vi "Run.vi"(8 "error in (no error)":errorcluster, 11 "LUnit Test Case V2 in":refnum<class "LUnit Test Case V2.lvclass">) -> (0 "error out":errorcluster, 2 "Results":T1[](array[typedef]))   [LabVIEW 2020, in "LUnit Test Case V2.lvclass"]
uses:
  LUnit Test Case V2.lvclass
  Result/Result.ctl
  Result/Status.ctl
  Result/Type.ctl
  LUnit Test Case V2.lvclass/LUnit Test Case V2.ctl
  Result/Result.lvlib
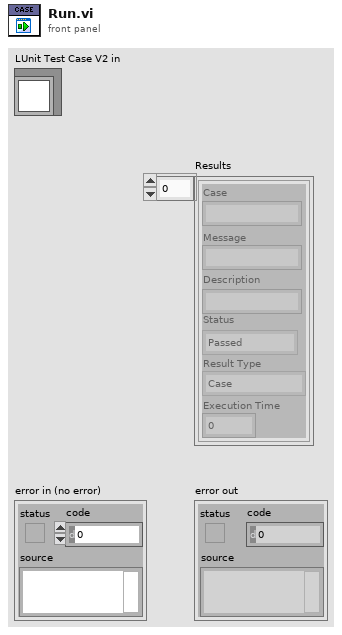
[diagram p1: front panel]
types:
  T1 = typedef "Result.lvlib/Result.ctl" = cluster{"Case":string, "Message":string, "Description":string, "Status":T2, "Result Type":T3, "Execution Time":dbl}
  T2 = typedef "Result.lvlib/Status.ctl" = enum16{"Passed", "Failed", "Error", "Skipped", "Setup Error", "Broken", "Teardown Error"}
  T3 = typedef "Result.lvlib/Type.ctl" = enum16{"Method", "Case", "Suite", "Pass", "Fail", "Skip", "Pass if", "Fail if", "Pass if Error", "Fail if Error", "Pass if Equal", "Fail if Equal"}
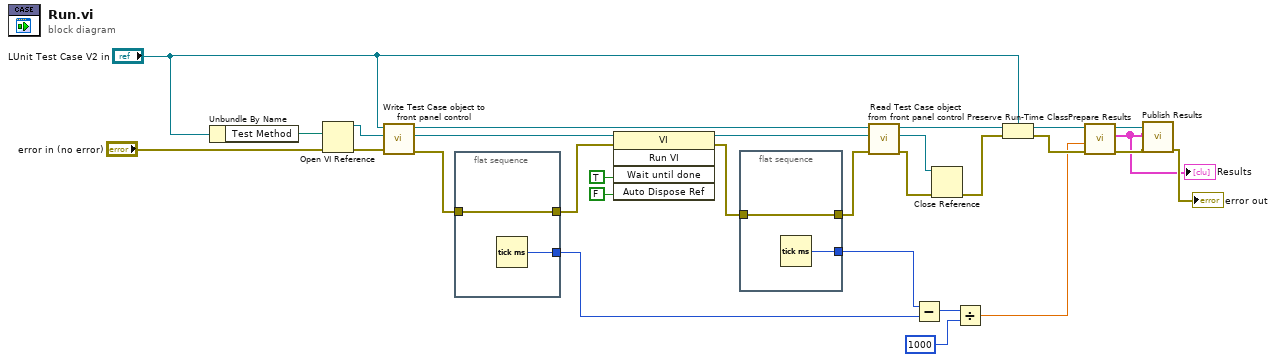
[diagram p0: block diagram]
diagram:
  n1 = Unbundle By Name("LUnit Test Case V2 in") -> ("Test Method"=w20:path)
  n2 = Open VI Reference(vi path=w20, error in (no error)="error in (no error)") -> (vi reference=w22:refnum<vi>, error out=w21:errorcluster)  [unwired: 4 in]
  n3 = call "Write Test Case object to front panel control.vi"("error in (no error)"=w21, "VI Refnum"=w22, "Test Case in"="LUnit Test Case V2 in") -> ("error out"=w13:errorcluster, "VI Refnum out"=w18:refnum<vi>, "Test Case out"=w15:refnum<class "LUnit Test Case V2.lvclass">)  [unwired: 6 in]
  n4 = flat-sequence {
    tunnel: w13 -> [w31]
    tunnel: [w31] -> w12
    tunnel: [w30] -> w8
    frame #0 {
      n5 = Tick Count (ms)() -> (millisecond timer value=w30:u32)
    }
  }
  n6 = invoke class="VI" method="Run VI"(reference=w18, error in=w12, "Wait until done"=TRUE ("Wait Until Done"), "Auto Dispose Ref"=FALSE ("Auto Dispose Reference")) -> (reference out=w19:refnum<vi>, error out=w11:errorcluster)  [unwired: 1 in, 3 out]
  n7 = flat-sequence {
    tunnel: w11 -> [w33]
    tunnel: [w33] -> w10
    tunnel: [w32] -> w9
    frame #0 {
      n8 = Tick Count (ms)() -> (millisecond timer value=w32:u32)
    }
  }
  n9 = call "Read Test Case object from front panel control.vi"("error in (no error)"=w10, "VI Refnum"=w19, "Test Case in"=w15) -> ("error out"=w24:errorcluster, "VI Refnum out"=w25:refnum<vi>, "Test Case out"=w23:refnum<class "LUnit Test Case V2.lvclass">)  [unwired: 6 in]
  n10 = Subtract(x=w9, y=w8) -> (x-y=w7:u32)
  n11 = Close Reference(reference=w25, error in (no error)=w24) -> (error out=w26:errorcluster)
  n12 = Divide(x=w7, y=u32 1000) -> (x/y=w5:dbl)
  n13 = Preserve Run-Time Class(object in=w23, error in=w26, 2:"LUnit Test Case V2 in") -> (object out=w14:refnum<class "LUnit Test Case V2.lvclass">, error out=w27:errorcluster)
  n14 = call "Prepare Results.vi"("error in (no error)"=w27, "Execution Time"=w5, "LUnit Test Case V2 in"=w14) -> ("error out"=w4:errorcluster, "Results"=w1:T1[], "LUnit Test Case V2 out"=w2:refnum<class "LUnit Test Case V2.lvclass">)  [unwired: 6 in]
  "Results" <- w1
  n15 = call "Publish Results.vi"("error in (no error)"=w4, "Results"=w1, "LUnit Test Case V2 In"=w2) -> ("error out"=→"error out":errorcluster)  [unwired: 7 in, 1 out]
